vi "Get Status.vi"(8 "error in (no error)":errorcluster, 11 "status":i32) -> (0 "error out":errorcluster, 2 "function return":u32, 3 "status out":i32)   [LabVIEW 2018, in "AndorSDK.lvlib"]
doc: "EXPNETTYPE unsigned int WINAPI GetStatus(int * status);"
uses:
  AndorSDK.lvlib
  ATMCD32D.dll
  OwnVIs/AndorOWN.lvlib
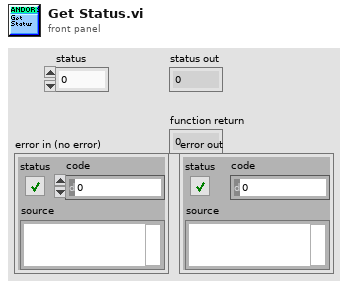
[diagram p1: front panel]
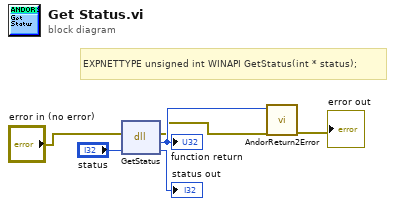
[diagram p0: block diagram]
diagram:
  # "EXPNETTYPE unsigned int WINAPI GetStatus(int * status);"
  n1 = dll-call lib="C:/Users/e14user/Documents/LabVIEW software/GitRepo/lib/ANDOR/Andor SDK/ATMCD32D.*" fn="GetStatus"(error in="error in (no error)", "status"="status") -> (error out=w2:errorcluster, w3:u32, "status"=→"status out":i32)  [unwired: 2 in, 1 out]
  "function return" <- w3
  n2 = call "AndorReturn2Error.vi"("error in (no error)"=w2, "Camera return"=w3) -> ("error out"=→"error out":errorcluster)  [unwired: 9 in]
